vi "Load Sub Panel.vi"(8 "error in":errorcluster, 10 "vi path":path) -> (0 "error out":errorcluster, 3 "vi reference out (strictly typed)":T1)   [LabVIEW 2021]
uses:
  <vilib>/myRIO/Common/Express VI Framework/typedefs/Config Pane Conn Pane Refnum.ctl
  <vilib>/myRIO/Common/Express VI Framework/typedefs/Timer Action.ctl
  <vilib>/Utility/miscctls.llb/LVPointTypeDef.ctl
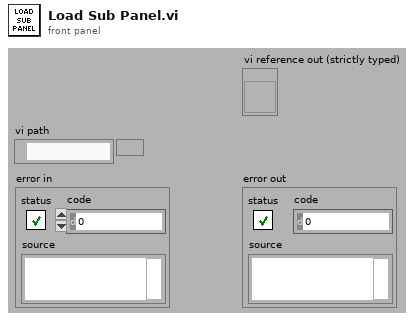
[diagram p1: front panel]
types:
  T1 = typedef "Config Pane Conn Pane Refnum.ctl" = refnum<vi>
  T2 = typedef "Timer Action.ctl" = enum16{"Start", "End", "Get All", "Clear All"}
  T3 = typedef "LVPointTypeDef.ctl" = cluster{"Horizontal":i16, "Vertical":i16}
  T4 = enum16{"Always On", "Always Off", "Off While Running"}
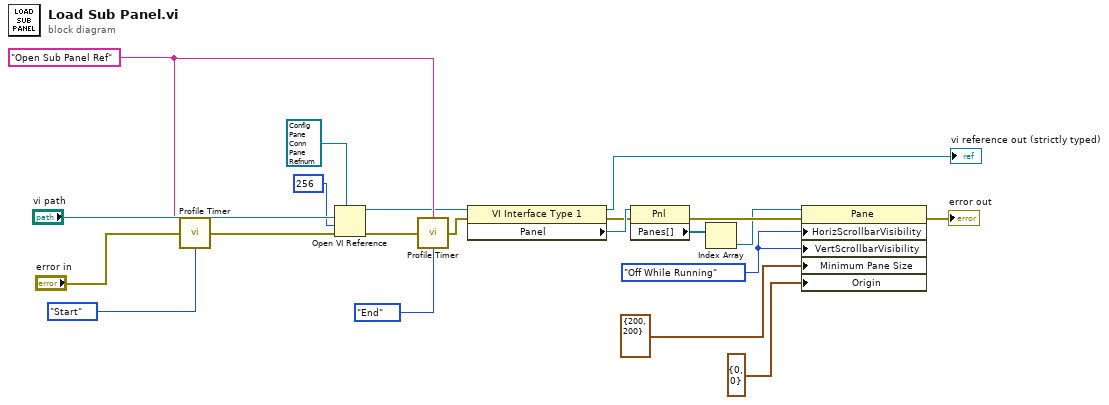
[diagram p0: block diagram]
diagram:
  w6 = "Open Sub Panel Ref" ("Label")
  w15 = T4."Off While Running" ("Horizontal Scrollbar Visibility")
  n1 = call <vilib>:"Profile Timer.vi"("Label"=w6, "error in (no error)"="error in", "Timer Action (Start)"=Timer_Action."Start") -> ("error out"=w11:errorcluster)  [unwired: 11 in, 1 out]
  n2 = Open VI Reference(type specifier VI Refnum (for type only)=T1 refnum ("Config Pane - Conn Pane Refum (for type only)"), vi path="vi path", options=256, error in (no error)=w11) -> (vi reference=w4:T1, error out=w10:errorcluster)  [unwired: 2 in]
  n3 = call <vilib>:"Profile Timer.vi"("Label"=w6, "error in (no error)"=w10, "Timer Action (Start)"=Timer_Action."End") -> ("error out"=w9:errorcluster)  [unwired: 11 in, 1 out]
  n4 = property class="VI Interface Type 1"(reference=w4, error in=w9) -> (reference out=→"vi reference out (strictly typed)":T1, error out=w17:errorcluster, "Panel"=w18:refnum<vi>)
  n5 = property class="Pnl"(reference=w18, error in=w17) -> (error out=w21:errorcluster, "Panes[]"=w19:refnum<vi>[])  [unwired: 1 out]
  n6 = Index Array(array=w19) -> (element=w20:refnum<vi>)  [unwired: 1 in]
  n7 = property on="Property Node" class="Pane"(reference=w20, error in=w21, "HorizScrollbarVisibility"=w15, "VertScrollbarVisibility"=w15, "Minimum Pane Size"=T3 {"Horizontal"=200, "Vertical"=200}, "Origin"=T3 {"Horizontal"=0, "Vertical"=0}) -> (error out=→"error out":errorcluster)  [unwired: 1 out]
